vi "Parse 14-2.vi"(11 "String":string) -> (3 "Puzzle":T1)   [LabVIEW 2020]
uses:
  Puzzle 14-2.ctl
  <vilib>/regexp/Match Regular Expression.xnode
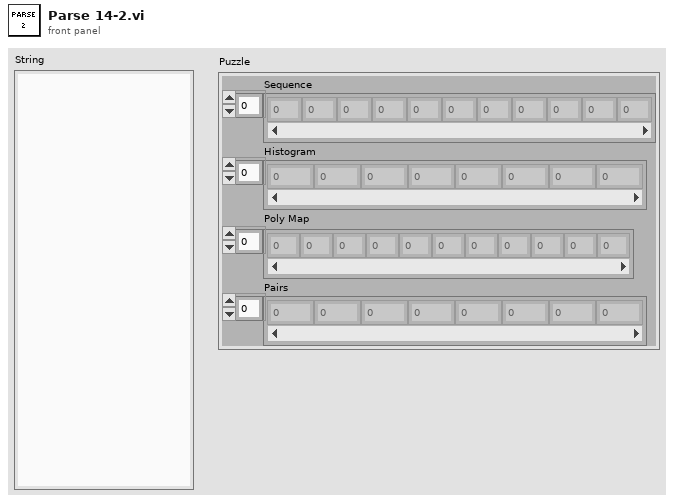
[diagram p1: front panel]
types:
  T1 = typedef "Puzzle 14-2.ctl" = cluster{"Sequence":u8[], "Histogram":i64[], "Poly Map":u8[], "Pairs":i64[]}
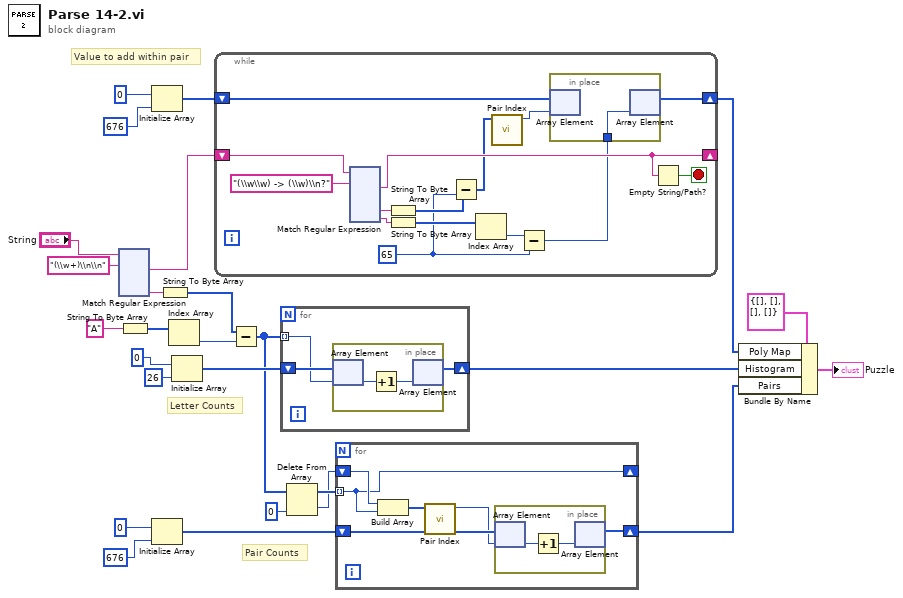
[diagram p0: block diagram]
diagram:
  # "Value to add within pair"
  # "Letter Counts"
  # "Pair Counts"
  n1 = xnode "Match Regular Expression"("input string"="String", "regular expression"="(\\w+)\\n\\n") -> ("after match"=w15:string, "submatch 1"=w25:string)  [unwired: 4 in, 4 out]
  n2 = String To Byte Array(string="A") -> (unsigned byte array=w23:u8[])
  n3 = Initialize Array(u8 0 ("element"), 676 ("dimension size")) -> (w10:u8[])
  n4 = Initialize Array(i64 0 ("element"), 676 ("dimension size")) -> (w6:i64[])
  n5 = String To Byte Array(string=w25) -> (unsigned byte array=w16:u8[])
  n6 = Index Array(array=w23) -> (element=w22:u8)  [unwired: 1 in]
  n7 = Initialize Array(i64 0, 26 ("dimension size")) -> (w19:i64[])
  n8 = while {
    shift-right: [w37] -> _
    shift-left: w15 -> [w41]
    shift-right: [w28] -> w9
    shift-left: w10 -> [w29]
    stop <- w36 stop-if-true
    w32 = u8 65 ("y")
    n9 = xnode "Match Regular Expression"("input string"=w41, "regular expression"="(\\w\\w) -> (\\w)\\n?") -> ("after match"=w37:string, "submatch 1"=w39:string, "submatch 2"=w38:string)  [unwired: 4 in, 4 out]
    n10 = String To Byte Array(string=w39) -> (unsigned byte array=w34:u8[])
    n11 = String To Byte Array(string=w38) -> (unsigned byte array=w35:u8[])
    n12 = Subtract(x=w34, y=w32) -> (x-y=w31:u8[])
    n13 = Index Array(array=w35) -> (element=w33:u8)  [unwired: 1 in]
    n14 = call "Pair Index.vi"("Pair"=w31) -> ("Index"=w30:i32)  [unwired: 10 in]
    n15 = Subtract(x=w33, y=w32) -> (x-y=w27:u8)
    n16 = in-place {
      in-place-border: w27 -> [w42]
      n17 = in-place-array #1(w29, w30) -> ()  [unwired: 1 out]
      n18 = in-place-array #1(w42) -> (w28:u8[])  [unwired: 1 out]
    }
    n19 = Empty String/Path?(string/path=w37) -> (empty?=w36:bool)
  }
  n20 = Subtract(x=w16, y=w22) -> (x-y=w5:u8[])
  n21 = for {
    tunnel: w5 -> [w161] mode=indexing
    shift-right: [w160] -> w17
    shift-left: w19 -> [w162]
    n22 = in-place {
      n23 = in-place-array #2(w162, w161) -> (w164:i64)
      n24 = Increment(x=w164) -> (x+1=w163:i64)
      n25 = in-place-array #2(w163) -> (w160:i64[])  [unwired: 1 out]
    }
  }
  n26 = Delete From Array(array=w5, index=0) -> (deleted portion=w3:u8, array with subset deleted=w4:u8[])  [unwired: 1 in]
  n27 = for {
    shift-right: [w165] -> w2
    shift-left: w6 -> [w167]
    tunnel: w4 -> [w169] mode=indexing
    shift-right: [w169] -> _
    shift-left: w3 -> [w170]
    n28 = Build Array(w170, w169) -> (w168:u8[])
    n29 = call "Pair Index.vi"("Pair"=w168) -> ("Index"=w166:i32)  [unwired: 10 in]
    n30 = in-place {
      n31 = in-place-array #3(w167, w166) -> (w172:i64)
      n32 = Increment(x=w172) -> (x+1=w171:i64)
      n33 = in-place-array #3(w171) -> (w165:i64[])  [unwired: 1 out]
    }
  }
  n34 = Bundle By Name(cluster=T1 {"Sequence"=[], "Histogram"=[], "Poly Map"=[], "Pairs"=[]} ("Puzzle"), "Poly Map"=w9, "Histogram"=w17, "Pairs"=w2) -> (→"Puzzle":T1)
